vi "Send Send Software Resume Trigger [RT].vi"(7 "Message Priority (Normal)":T1=enum."Normal", 8 "error in (no error)":errorcluster, 10 "Execute?":bool, 11 "Message Enqueuer":refnum<class "Message Enqueuer.lvclass">) -> (0 "error out":errorcluster, 3 "Message Enqueuer out":refnum<class "Message Enqueuer.lvclass">)   [LabVIEW 2015, in "CS++Fgen.lvlib" / "Send Software Resume Trigger [RT] Msg.lvclass"]
doc: "Sends the <B>CS++Fgen.lvlib:Send Software Resume Trigger [RT] Msg.lvclass</B> message.\n\n<B>CS++Fgen.lvlib:CS++Fgen.lvclass:Send Software Resume Trigger [RT].vi</B> Description:\n\nThis VI sends a software-generated resume trigger to the function generator. If the trigger source is not set to software trigger, this VI returns the error IVIFGEN_ERROR_TRIGGER_NOT_SOFTWARE.\n\nNotes:\n\n(1) This VI does not normally check the instrument status. Typically, you call this VI only in a sequence of calls to other low-level driver VIs. The sequence performs one operation. You use the low-level VIs to optimize one or more aspects of interaction with the instrument. If you want to check the instrument status, call the IviFgen Error-Query VI at the conclusion of the sequence.\n\n(2) This VI is part of the IviFgenResumeTrigger [RT] extension group."
uses:
  Send Software Resume Trigger [RT] Msg.lvclass
  <vilib>/ActorFramework/Message Enqueuer/Message Enqueuer.lvclass
  <vilib>/ActorFramework/Message Enqueuer/Message Priority.ctl
  Send Software Resume Trigger [RT] Msg.lvclass/Send Software Resume Trigger [RT] Msg.ctl
  <vilib>/ActorFramework/Message Enqueuer/Message Enqueuer.lvclass/Message Enqueuer.ctl
  <vilib>/ActorFramework/Message Priority Queue/Priority Enqueue.vi
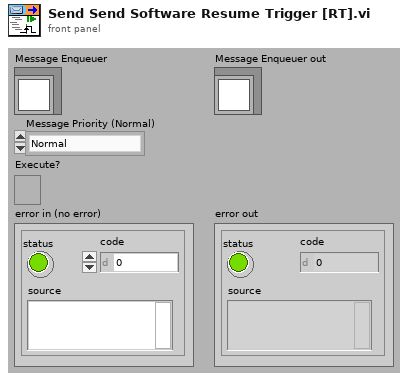
[diagram p1: front panel]
types:
  T1 = typedef "Actor Framework.lvlib/Message Enqueuer.lvclass/Message Priority.ctl" = enum16{"Low", "Normal", "High"}
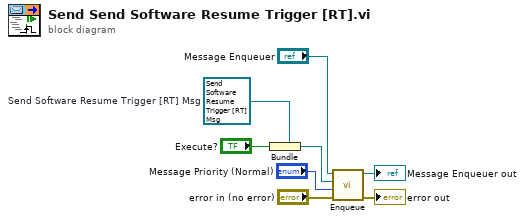
[diagram p0: block diagram]
diagram:
  w2 = refnum<class "Send Software Resume Trigger [RT] Msg.lvclass"> refnum  # Send Software Resume Trigger [RT] Msg
  n1 = Bundle(cluster=w2, "Execute?") -> (w5:refnum<class "Send Software Resume Trigger [RT] Msg.lvclass">)
  n2 = call <vilib>:"Enqueue.vi"("error in (no error)"="error in (no error)", "Message Priority (Normal)"="Message Priority (Normal)", "Message"=w5, "Message Enqueuer in"="Message Enqueuer") -> ("error out"=→"error out":errorcluster, "Message Enqueuer out"=→"Message Enqueuer out":refnum<class "Message Enqueuer.lvclass">)  [unwired: 6 in]
